vi "Ballard 1553 - Initialize - RTs Only Checking.vi"(11 "channels":T1[](array[typedef]) {"RTs"."Mode Codes"."Words Item Refs" format="%.0x"; "RTs"."Mode Codes"."Timestamp Channel Data Reference" format="%.0x"; "RTs"."subAddresses"."Words Item Refs" format="%.0x"; "RTs"."subAddresses"."Timestamp Channel Data Reference" format="%.0x"; "RTs"."Status Channel Data Reference" format="%.0x"; "RTs"."Command Channels Refs" format="%.0x"; "BC"."Acyclic Frames Trigger Channels Refs" format="%.0x"; "BC"."Command Channels Refs" format="%.0x"; "BC"."messages"."Timestamp Channel Data Reference" format="%.0x"; "BC"."messages"."Status Channel Data Refs" format="%.0x"; "BC"."messages"."Words Item Refs" format="%.0x"; "BC"."messages"."Words Block Data Refs"."Data Reference" format="%.0x"}) -> (3 "RTs Only?":bool)   [LabVIEW 2017, in "Ballard MIL-1553 Engine.lvlib"]
doc: "This VI checks whether it's a RTs only configuration (no BC present for any Channel).\nWe consider that there is no BC when there are no Messages configured."
uses:
  Ballard MIL-1553 Engine.lvlib
  Shared/Controls and Global/RT Channel.ctl
  Shared/Controls and Global/RT BC.ctl
  <vilib>/NI Veristand/Custom Device API/Custom Device Item Ref.ctl
  Shared/Controls and Global/RT Message.ctl
  Shared/Controls and Global/RT messageType.ctl
  Shared/Controls and Global/RT CWD1.ctl
  Shared/Controls and Global/RT CWD2.ctl
  <vilib>/NI Veristand/Custom Device API/Data Reference.ctl
  <vilib>/NI Veristand/Custom Device API/Block Data Reference.ctl
  Shared/Controls and Global/RT Remote Terminal.ctl
  Shared/Controls and Global/RT Remote Terminal_rtMode.ctl
  Shared/Controls and Global/RT Remote Terminal_RT subAddress.ctl
  Shared/Controls and Global/RT Remote Terminal_RT direction.ctl
  Shared/Controls and Global/RT Remote Terminal_RT Mode Code.ctl
  <vilib>/NI VeriStand/Custom Device API/Custom Device API.lvlib
  Shared/Ballard 1553 Shared.lvlib
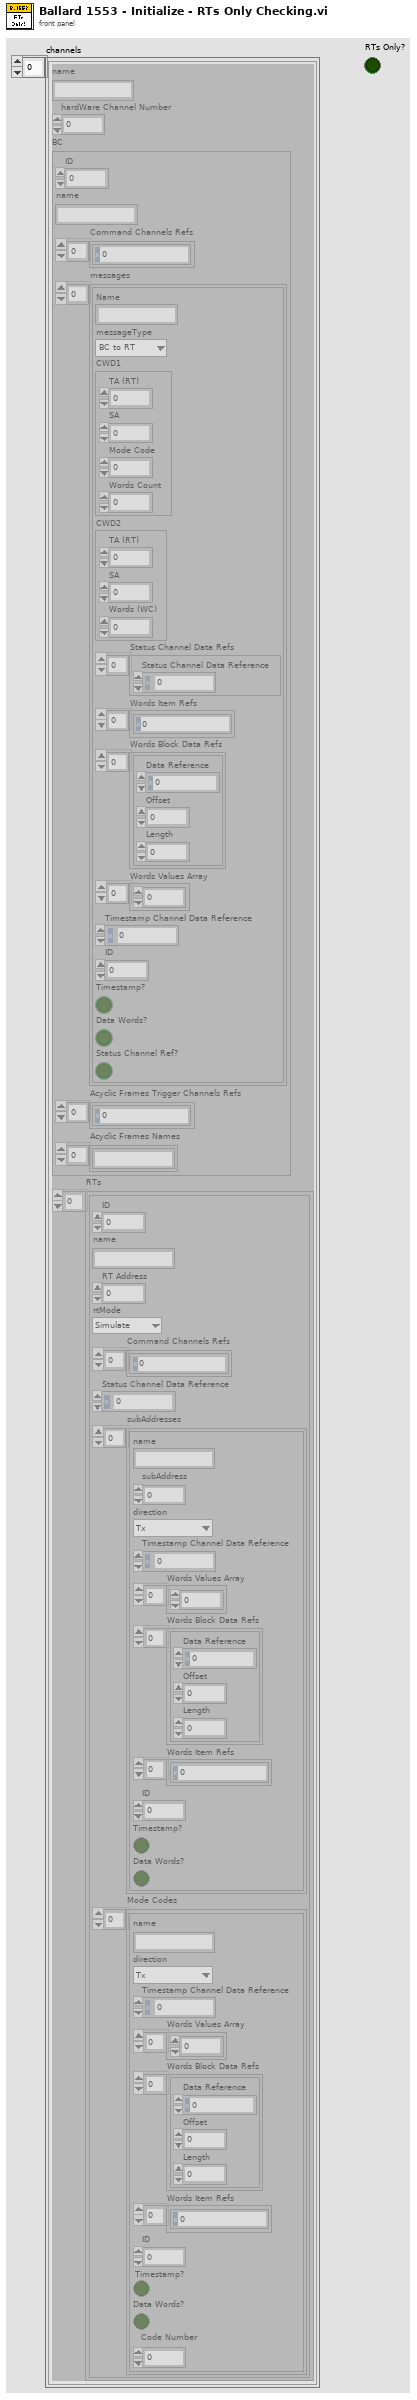
[diagram p1: front panel]
types:
  T1 = typedef "Ballard 1553 Shared.lvlib/RT Channel.ctl" = cluster{"name":string, "hardWare Channel Number":u16, "BC":T2, "RTs":T10[]}
  T2 = typedef "Ballard 1553 Shared.lvlib/RT BC.ctl" = cluster{"ID":i32, "name":string, "Command Channels Refs":T3[], "messages":T4[], "Acyclic Frames Trigger Channels Refs":T3[], "Acyclic Frames Names":string[]}
  T3 = typedef "Custom Device API.lvlib/Custom Device Item Ref.ctl" = u64
  T4 = typedef "Ballard 1553 Shared.lvlib/RT Message.ctl" = cluster{"Name":string, "messageType":T5, "CWD1":T6, "CWD2":T7, "Status Channel Data Refs":T8[], "Words Item Refs":T3[], "Words Block Data Refs":T9[], "Words Values Array":u16[], "Timestamp Channel Data Reference":T8, "ID":i32, "Timestamp?":bool, "Data Words?":bool, "Status Channel Ref?":bool}
  T5 = typedef "Ballard 1553 Shared.lvlib/RT messageType.ctl" = enum16{"BC to RT", "RT to BC", "RT to RT", "MC (Rx)", "MC (Tx)"}
  T6 = typedef "Ballard 1553 Shared.lvlib/RT CWD1.ctl" = cluster{"TA (RT)":i8, "SA":i8, "Mode Code":i8, "Words Count":i8}
  T7 = typedef "Ballard 1553 Shared.lvlib/RT CWD2.ctl" = cluster{"TA (RT)":i8, "SA":i8, "Words (WC)":i8}
  T8 = typedef "Custom Device API.lvlib/Data Reference.ctl" = i32
  T9 = typedef "Custom Device API.lvlib/Block Data Reference.ctl" = cluster{"Data Reference":T8, "Offset":u64, "Length":u64}
  T10 = typedef "Ballard 1553 Shared.lvlib/RT Remote Terminal.ctl" = cluster{"ID":i32, "name":string, "RT Address":i32, "rtMode":T11, "Command Channels Refs":T3[], "Status Channel Data Reference":T8, "subAddresses":T12[], "Mode Codes":T14[]}
  T11 = typedef "Ballard 1553 Shared.lvlib/RT Remote Terminal_rtMode.ctl" = enum16{"Simulate", "Monitor", "Disable"}
  T12 = typedef "Ballard 1553 Shared.lvlib/RT Remote Terminal_RT subAddress.ctl" = cluster{"name":string, "subAddress":i8, "direction":T13, "Timestamp Channel Data Reference":T8, "Words Values Array":u16[], "Words Block Data Refs":T9[], "Words Item Refs":T3[], "ID":i32, "Timestamp?":bool, "Data Words?":bool}
  T13 = typedef "Ballard 1553 Shared.lvlib/RT Remote Terminal_RT direction.ctl" = enum16{"Tx", "Rx"}
  T14 = typedef "Ballard 1553 Shared.lvlib/RT Remote Terminal_RT Mode Code.ctl" = cluster{"name":string, "direction":T13, "Timestamp Channel Data Reference":T8, "Words Values Array":u16[], "Words Block Data Refs":T9[], "Words Item Refs":T3[], "ID":i32, "Timestamp?":bool, "Data Words?":bool, "Code Number":i32}
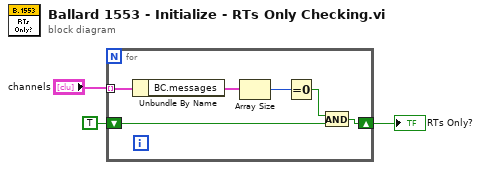
[diagram p0: block diagram]
diagram:
  n1 = for {
    tunnel: "channels" -> [w9] mode=indexing
    shift-right: [w4] -> w1
    shift-left: TRUE -> [w5]
    n2 = Unbundle By Name(w9) -> ("BC.messages"=w8:T4[])
    n3 = Array Size(array=w8) -> (size(s)=w7:i32)
    n4 = Equal To 0?(x=w7) -> (x = 0?=w6:bool)
    n5 = And(x=w6, y=w5) -> (x .and. y?=w4:bool)
  }
  "RTs Only?" <- w1
